vi "9_SubroutineTests.vi"() -> ()   [LabVIEW 2012]
uses:
  <userlib>/BotSpeak/VIs/Scripting/URAPI_WriteDigitalOut_num.vi
  <userlib>/BotSpeak/VIs/Scripting/URAPI_Delay_num.vi
  <userlib>/BotSpeak/VIs/Scripting/URAPI_WriteAnalogOut.vi
  <userlib>/BotSpeak/VIs/Scripting/URAPI_ForStart_num.vi
panel:
  out "BotSpeak":string="SET var,0\nSET Sub1_return,0\nSET sub2_start,0\nSET Sub1_start,0\nSCRIPT\nSET AO[0],1\nSET count0,0\nIF ~(count0 > 1) GOTO 9\nSET Sub1_return,HERE\nADD Sub1_return,13\nGOTO 21\nADD count0,1\nIF (count0 < 5) GOTO 4\nSET test,END\nend\nSET sub2_start,HERE\nSET DIO[13],1\nWAIT 0.500000\nSET DIO[13],0\nWAIT 0.500000\nGOTO sub2_return\nSET Sub1_start,HERE\nSET DIO[13],1\nWAIT 0.500000\nSET DIO[13],0\nWAIT 0.500000\nGOTO Sub1_return\nENDSCRIPT\nRUN&WAIT sub2_start\nRUN&WAIT Sub1_start\nRUN&WAIT 0\nGET test\n"
  out "expected response":string="0\r\n0\r\n0\r\n0\r\nstart script\r\nend script\r\n..............................................\nDone\r\n..........\nDone\r\n..............................................\nDone\r\n98\r\n"
  out "response":string="0\r\n0\r\n0\r\n0\r\nstart script\r\nend script\r\n..............................................\nDone\r\n..........\nDone\r\n..............................................\nDone\r\n98\r\n"
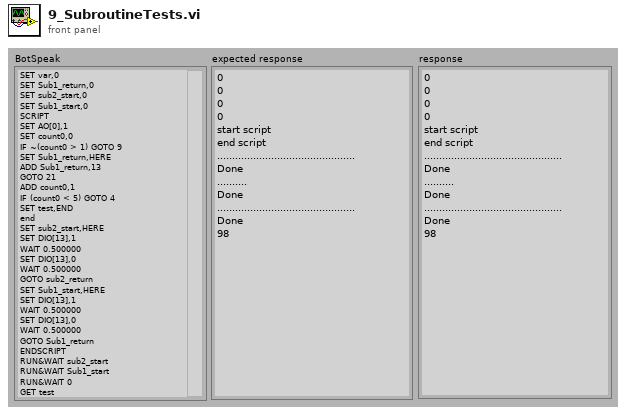
[diagram p1: front panel]
types:
  T1 = typedef "URAPI_Control.ctl" = cluster{"Script":string, "Whiles":u8[], "Ifs":u8[], "Supress Err":bool, "Errors":string}
  T2 = typedef "BotSpeak_Control.ctl" = cluster{"Address":string, "Reply EOF":string, "Hardware":path, "Retries":i8, "Timeout":i32}
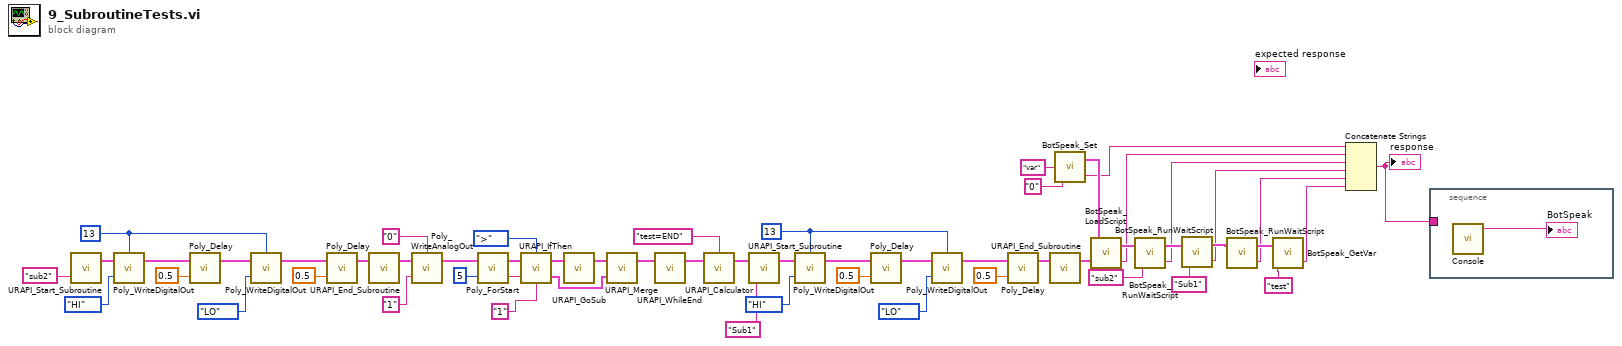
[diagram p0: block diagram]
diagram:
  w16 = u8 13 ("Channel")
  w28 = u8 13 ("Channel")
  n1 = call <userlib>:"URAPI_Start_Subroutine.vi"("Subroutine Name"="sub2") -> ("URAPI Script out"=w6:T1)  [unwired: 2 in]
  n2 = call-poly <userlib>:"Poly_WriteDigitalOut.vi"("Value"=enum16{"LO", "HI"}."HI" ("Variable In"), "URAPI Script"=w6, "Channel"=w16) -> ("URAPI Script"=w8:T1)  [unwired: 1 in, 1 out]
  n3 = call-poly <userlib>:"Poly_Delay.vi"("Time In"=sgl 0.5, "URAPI Script"=w8) -> ("URAPI Script out"=w14:T1)  [unwired: 3 in]
  n4 = call-poly <userlib>:"Poly_WriteDigitalOut.vi"("Value"=enum16{"LO", "HI"}."LO" ("Variable In"), "URAPI Script"=w14, "Channel"=w16) -> ("URAPI Script"=w13:T1)  [unwired: 1 in, 1 out]
  n5 = call-poly <userlib>:"Poly_Delay.vi"("Time In"=sgl 0.5, "URAPI Script"=w13) -> ("URAPI Script out"=w15:T1)  [unwired: 3 in]
  n6 = call <userlib>:"URAPI_End_Subroutine.vi"("URAPI Script in"=w15) -> ("URAPI Script out"=w7:T1)  [unwired: 2 in]
  n7 = call-poly <userlib>:"Poly_WriteAnalogOut.vi"("Variable In"="1" ("String"), "URAPI Script"=w7, "Channel"="0") -> ("URAPI Script"=w27:T1)  [unwired: 1 in, 1 out]
  n8 = call-poly <userlib>:"Poly_ForStart.vi"("Iterations"=u8 5, "URAPI Script"=w27) -> ("variable"=w21:string, "URAPI Script Out"=w24:T1)  [unwired: 2 in]
  n9 = call <userlib>:"URAPI_IfThen.vi"("Variable In"=w21, "Compare to"="1", "URAPI Script"=w24, "Comparison"=enum16{">", "<", "=", "!="}.">") -> ("URAPI False"=w17:T1, "URAPI True"=w23:T1)
  n10 = call <userlib>:"URAPI_GoSub.vi"("URAPI Script"=w23) -> ("URAPI Script out"=w19:T1)  [unwired: 2 in]
  n11 = call <userlib>:"URAPI_Merge.vi"("URAPI False"=w17, "URAPI True"=w19) -> ("URAPI Script"=w18:T1)  [unwired: 3 in]
  n12 = call <userlib>:"URAPI_WhileEnd.vi"("URAPI Script"=w18) -> ("URAPI Script Out"=w25:T1)  [unwired: 4 in]
  n13 = call <userlib>:"URAPI_Calculator.vi"("URAPI Script"=w25, "Formula"="test=END") -> ("URAPI Script"=w29:T1)  [unwired: 2 in, 1 out]
  n14 = call <userlib>:"URAPI_Start_Subroutine.vi"("Subroutine Name"="Sub1", "URAPI Script"=w29) -> ("URAPI Script out"=w34:T1)  [unwired: 1 in]
  n15 = call-poly <userlib>:"Poly_WriteDigitalOut.vi"("Value"=enum16{"LO", "HI"}."HI" ("Variable In"), "URAPI Script"=w34, "Channel"=w28) -> ("URAPI Script"=w41:T1)  [unwired: 1 in, 1 out]
  n16 = call-poly <userlib>:"Poly_Delay.vi"("Time In"=sgl 0.5, "URAPI Script"=w41) -> ("URAPI Script out"=w35:T1)  [unwired: 3 in]
  n17 = call-poly <userlib>:"Poly_WriteDigitalOut.vi"("Value"=enum16{"LO", "HI"}."LO" ("Variable In"), "URAPI Script"=w35, "Channel"=w28) -> ("URAPI Script"=w36:T1)  [unwired: 1 in, 1 out]
  n18 = call-poly <userlib>:"Poly_Delay.vi"("Time In"=sgl 0.5, "URAPI Script"=w36) -> ("URAPI Script out"=w31:T1)  [unwired: 3 in]
  n19 = call <userlib>:"URAPI_End_Subroutine.vi"("URAPI Script in"=w31) -> ("URAPI Script out"=w4:T1)  [unwired: 2 in]
  n20 = call <userlib>:"BotSpeak_Set.vi"("value"="0", "Variable In"="var") -> ("response"=w42:string, "Bot Settings"=w43:T2)  [unwired: 1 in]
  n21 = call <userlib>:"BotSpeak_LoadScript.vi"("URAPI Script"=w4, "Bot Settings"=w43) -> ("total response"=w49:string, "Bot Settings"=w54:T2)
  n22 = call <userlib>:"BotSpeak_RunWaitScript.vi"("Subroutine (runs prgm if unwired)"="sub2", "Bot Settings"=w54) -> ("response"=w48:string, "Bot Settings"=w53:T2)
  n23 = call <userlib>:"BotSpeak_RunWaitScript.vi"("Subroutine (runs prgm if unwired)"="Sub1" ("Variable In"), "Bot Settings"=w53) -> ("response"=w47:string, "Bot Settings"=w51:T2)
  n24 = call <userlib>:"BotSpeak_RunWaitScript.vi"("Bot Settings"=w51) -> ("response"=w46:string, "Bot Settings"=w50:T2)  [unwired: 1 in]
  n25 = call <userlib>:"BotSpeak_GetVar.vi"("Variable In"="test", "Bot Settings"=w50) -> ("value"=w45:string)  [unwired: 1 out]
  n26 = Concatenate Strings(w42, w49, w48, w47, w46, w45) -> (w44:string)
  "response" <- w44
  n27 = stacked-sequence {
    tunnel: w44 -> [_]
    frame #0 {
      n28 = call <userlib>:"Console.vi"() -> ("BotSpeak"=→"BotSpeak":string)  [unwired: 4 in, 1 out]
    }
  }
